vi "Scale Voltage.vi"(1 "Scale factor":dbl min=-2.0 max=2.0, 2 "Breakdown Low":dbl=-0.03, 3 "Breakdown High":dbl=0.1) -> (0 "Real Voltage":dbl=0.035)   [LabVIEW 2011]
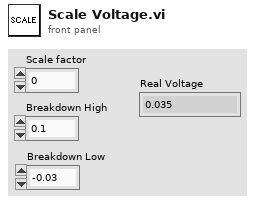
[diagram p1: front panel]
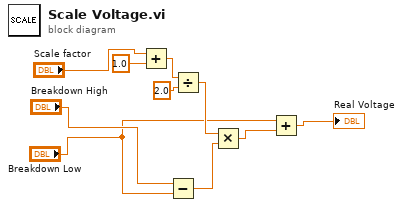
[diagram p0: block diagram]
diagram:
  n1 = Add(x="Scale factor", y=1.0) -> (x+y=w6:dbl)
  n2 = Subtract(x="Breakdown High", y="Breakdown Low") -> (x-y=w4:dbl)
  n3 = Divide(x=w6, y=2.0) -> (x/y=w5:dbl)
  n4 = Multiply(x=w5, y=w4) -> (x*y=w3:dbl)
  n5 = Add(x="Breakdown Low", y=w3) -> (x+y=→"Real Voltage":dbl)
